vi "Ex6.vi"() -> ()   [LabVIEW 2016]
uses:
  <vilib>/Analysis/polynomials.llb/Unique Numbers and Multiplicity (DBL).vi
  <vilib>/Analysis/NI_AALPro.lvlib
panel:
  out "발생":dbl[](array[numeric])
  out "결과":string
  in  "N":dbl
  out "Unique Numbers":dbl[](array[numeric]) caption="중복을 제외한 랜덤 넘버" format="%#.6g"
  out "Sorting":dbl[](array[numeric])
  # "번째 큰수:"
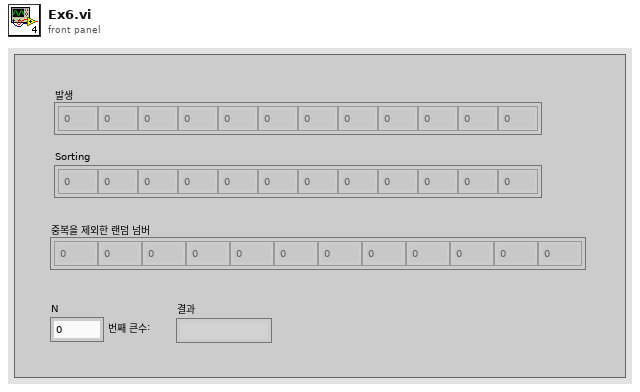
[diagram p1: front panel]
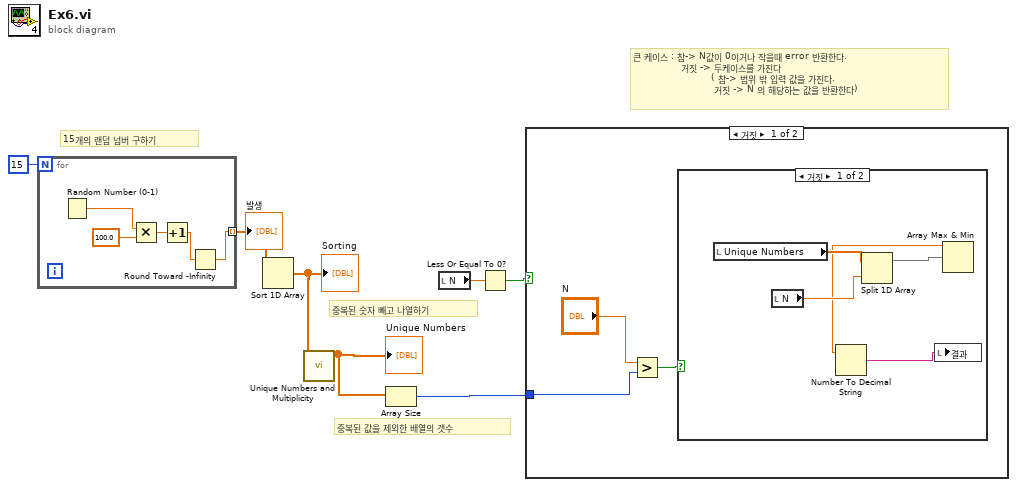
[diagram p0: block diagram]
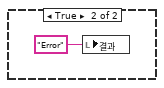
[diagram p2: hidden frame]
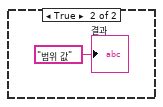
[diagram p3: hidden frame]
diagram:
  # "큰 케이스 : 참-> N값이 0이거나 작을때 error 반환한다.\n                거짓 -> 두케이스를 가진다 \n                          ( 참-> 범위 밖 입력 값을 가진다.\n                           거짓 -> N 의 해당하는 값을 반환한다)"
  # "중복된 값을 제외한 배열의 갯수"
  # "15개의 랜덤 넘버 구하기"
  # "중복된 숫자 빼고 나열하기"
  n1 = for {
    N: 15 -> [_]
    tunnel: [w8] -> w6 mode=indexing
    n2 = Random Number (0-1)() -> (number: 0 to 1=w12:dbl)
    n3 = Multiply(x=w12, y=100.0) -> (x*y=w10:dbl)
    n4 = Increment(x=w10) -> (x+1=w9:dbl)
    n5 = Round Toward -Infinity(1:w9) -> (0:w8:dbl)
  }
  "발생" <- w6
  n6 = Sort 1D Array(array=w6) -> (sorted array=w5:dbl[])
  "Sorting" <- w5
  n7 = call-poly <vilib>:"Unique Numbers and Multiplicity.vi"("Numbers"=w5) -> ("Unique Numbers"=w4:dbl[])  [unwired: 8 in, 2 out]
  "Unique Numbers" <- w4
  n8 = Array Size(array=w4) -> (size(s)=w1:i32)
  n9 = local read "N"() -> (w3:dbl)
  n10 = Less Or Equal To 0?(x=w3) -> (x <= 0?=w2:bool)
  n11 = case shown="거짓" w2 {
    tunnel: w1 -> [w13 _]
    frame False {
      n12 = Greater?(x="N", y=w13) -> (0:w15:bool)
      n13 = case shown="거짓" w15 {
        frame False {
          n14 = local read "Unique Numbers"() -> (w20:dbl[])
          n15 = local read "N"() -> (w19:dbl)
          n16 = Split 1D Array(array=w20, index=w19) -> (first subarray=w18:dbl[])  [unwired: 1 out]
          n17 = Array Max & Min(array=w18) -> (max value=w17:dbl)  [unwired: 3 out]
          n18 = Number To Decimal String(number=w17) -> (decimal integer string=w16:string)  [unwired: 1 in]
          n19 = local write "결과"(w16) -> ()
        }
        frame True {
          n20 = local write "결과"("Error" ("문자열")) -> ()
        }
      }
    }
    frame True {
      "결과" <- "범위 값" ("문자열")
    }
  }
